vi "Read Time.vi"(11 "Debug Data in":refnum<class "Debug Data.lvclass">) -> (2 "Time":dbl, 3 "Debug Data out":refnum<class "Debug Data.lvclass">)   [LabVIEW 2020, in "Debug Data.lvclass"]
uses:
  Debug Data.lvclass
  Debug Data.lvclass/Debug Data.ctl
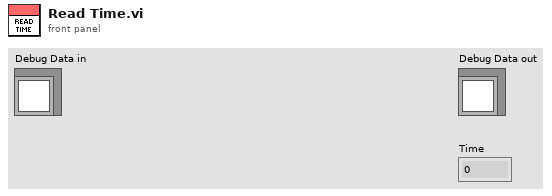
[diagram p1: front panel]
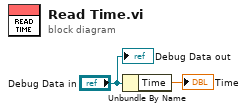
[diagram p0: block diagram]
diagram:
  n1 = Unbundle By Name("Debug Data in") -> ("Time"=→"Time":dbl)
  "Debug Data out" <- "Debug Data in"
